vi "update t0.vi"(11 "Template in":refnum<class "Template.lvclass">) -> (2 "t0":timestamp, 3 "Template out":refnum<class "Template.lvclass">)   [LabVIEW 2020, in "Template.lvlib" / "Template.lvclass"]
uses:
  Template.lvclass
  Template.lvclass/Template.ctl
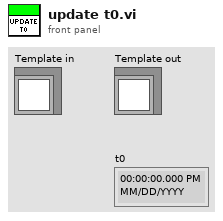
[diagram p1: front panel]
types:
  T1 = typedef "Template.lvlib/Template.lvclass/daq params.ctl" = cluster{"t0":timestamp, "Reset t0":refnum<notifier>}
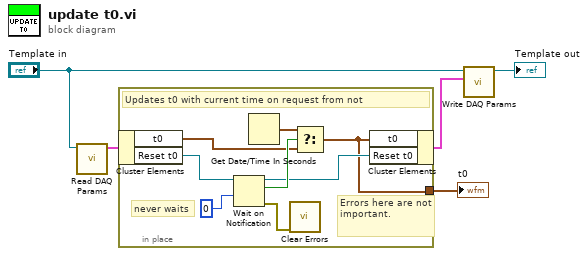
[diagram p0: block diagram]
diagram:
  n1 = call "Read DAQ Params.vi"("Template in"="Template in") -> ("DAQ Params"=w4:T1)  [unwired: 10 in]
  n2 = in-place {
    in-place-border: [w6] -> w1
    # "Errors here are not important."
    # "never waits"
    # "Updates t0 with current time on request from not"
    n3 = in-place-cluster #1(w4) -> ("t0"=w9:timestamp, "Reset t0"=w8:refnum<notifier>)
    n4 = Wait on Notification(notifier=w8, timeout in ms (-1)=0) -> (notifier out=w7:refnum<notifier>, notification=w11:bool, error out=w12:errorcluster)  [unwired: 2 in, 1 out]
    n5 = Get Date/Time In Seconds() -> (seconds since 1Jan1904=w10:timestamp)
    n6 = call <vilib>:"Clear Errors.vi"("error in (no error)"=w12) -> ()  [unwired: 5 in, 2 out]
    n7 = Select(t=w10, s=w11, f=w9) -> (s? t:f=w6:timestamp)
    n8 = in-place-cluster #1("t0"=w6, "Reset t0"=w7) -> (w5:T1)
  }
  "t0" <- w1
  n9 = call "Write DAQ Params.vi"("DAQ Params"=w5, "Template in"="Template in") -> ("Template out"=→"Template out":refnum<class "Template.lvclass">)  [unwired: 9 in]
